vi "Pic Overlay Basic Point.vi"(8 "error in (no error)":errorcluster, 10 "Picture in":picture, 11 "LF2R IDE in":refnum<class "Main Panel.lvclass">) -> (0 "error out":errorcluster, 2 "Picture out":picture, 3 "LF2R IDE out":refnum<class "Main Panel.lvclass">)   [LabVIEW 2018, in "Main Panel.lvlib" / "Main Panel.lvclass"]
uses:
  Main Panel.lvclass
  Main Panel.lvclass/Main Panel.ctl
  Picture Process/Picture Process.lvclass
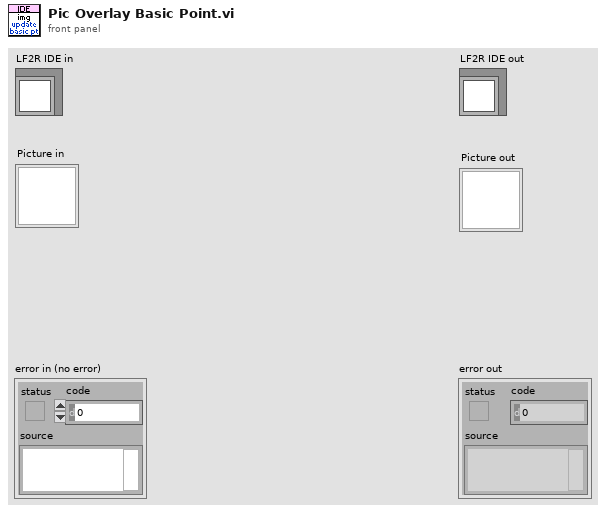
[diagram p1: front panel]
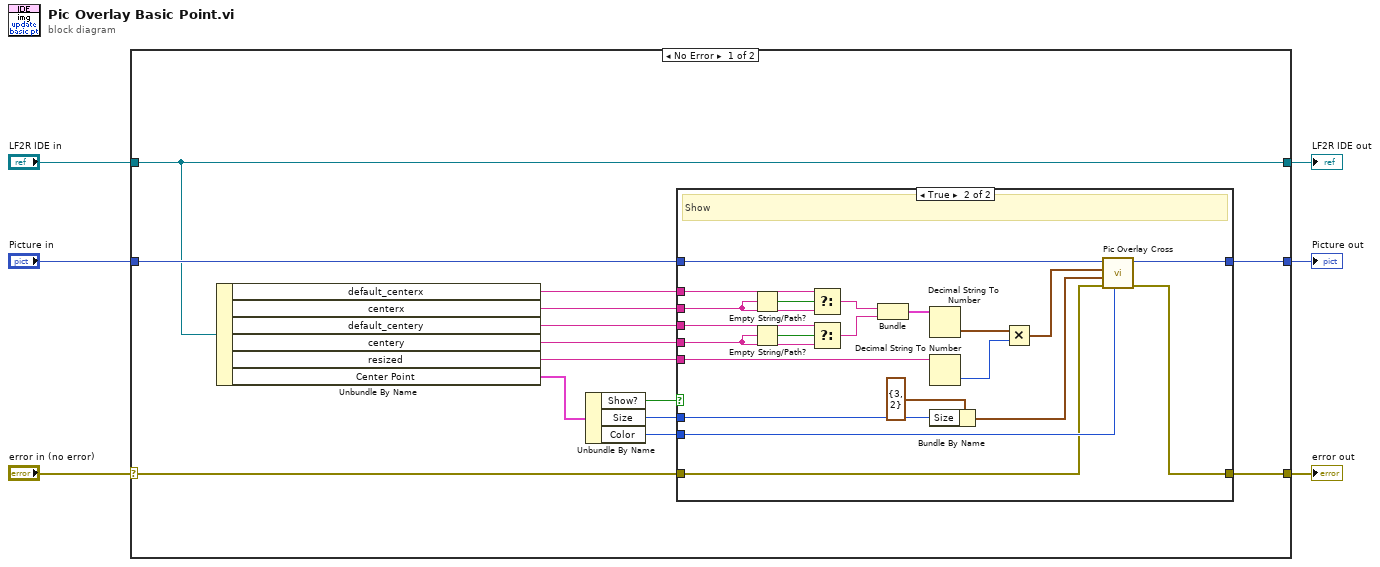
[diagram p0: block diagram]
diagram:
  n1 = case shown="No Error" "error in (no error)" {
    selector: "error in (no error)" -> [w8 w46]
    tunnel: [w7 w46] -> w5
    tunnel: [w9 w45] -> w3
    tunnel: "LF2R IDE in" -> [w9 w45]
    tunnel: "Picture in" -> [w11 w44]
    tunnel: [w10 w44] -> w1
    frame No Error {
      n2 = Unbundle By Name(w9) -> ("default_centerx"=w19:string, "centerx"=w18:string, "default_centery"=w17:string, "centery"=w16:string, "resized"=w20:string, "Center Point"=w15:cluster{"Size":i32, "Color":u32, "Show?":bool})
      n3 = Unbundle By Name(w15) -> ("Show?"=w14:bool, "Size"=w13:i32, "Color"=w12:u32)
      n4 = case shown="True" w14 {
        tunnel: w20 -> [_ w43]
        tunnel: w19 -> [_ w39]
        tunnel: w18 -> [_ w38]
        tunnel: w17 -> [_ w36]
        tunnel: w16 -> [_ w35]
        tunnel: w13 -> [_ w28]
        tunnel: w12 -> [_ w30]
        tunnel: w11 -> [w22 w26]
        tunnel: [w22 w25] -> w10
        tunnel: w8 -> [w21 w24]
        tunnel: [w21 w23] -> w7
        frame False {
          # "Skip"
        }
        frame True {
          # "Show"
          n5 = Empty String/Path?(string/path=w38) -> (empty?=w40:bool)
          n6 = Empty String/Path?(string/path=w35) -> (empty?=w37:bool)
          n7 = Select(t=w39, s=w40, f=w38) -> (s? t:f=w34:string)
          n8 = Select(t=w36, s=w37, f=w35) -> (s? t:f=w33:string)
          n9 = Bundle("centerx"=w34, "centery"=w33) -> (w32:cluster{"centerx":string, "centery":string})  [unwired: 1 in]
          n10 = Decimal String To Number(string=w32) -> (number=w42:cluster{"centerx":i32, "centery":i32})  [unwired: 2 in, 1 out]
          n11 = Decimal String To Number(string=w43) -> (number=w41:i32)  [unwired: 2 in, 1 out]
          n12 = Bundle By Name(cluster=cluster{"Size":i32, "Width":u16} {"Size"=3, "Width"=2} ("Line"), "Size"=w28) -> (w27:cluster{"Size":i32, "Width":u16})
          n13 = Multiply(x=w42, y=w41) -> (x*y=w31:cluster{"centerx":i32, "centery":i32})
          n14 = call "Pic Overlay Cross.vi"("Color"=w30, "error in (no error)"=w24, "Line"=w27, "Position"=w31, "Picture in"=w26) -> ("error out"=w23:errorcluster, "Picture out"=w25:picture)  [unwired: 5 in]
        }
      }
    }
    frame Error {
    }
  }
  "error out" <- w5
  "LF2R IDE out" <- w3
  "Picture out" <- w1
